vi "Publish (Raw Payload).vi"(4 "timeout (1000ms)":i32=1000, 5 "RETAIN":bool, 6 "QoS":T1, 7 "DUP (Re-delivery attempt)":bool, 8 "error in (no error)":errorcluster, 9 "Binary Payload":u8[](array[numeric]) format="%08b", 10 "Topic Name":string, 11 "Client in":refnum<class "Client.lvclass">) -> (0 "error out":errorcluster, 2 "Published":bool, 3 "Client out":refnum<class "Client.lvclass">)   [LabVIEW 2013, in "MQTT Client.lvlib" / "Client.lvclass"]
uses:
  Client.lvclass
  <vilib>/LabVIEW Open Source Project/MQTT Control Packets/Control Packets/ControlPacket/QualityOfService -- enum.ctl
  <vilib>/LabVIEW Open Source Project/MQTT Control Packets/Control Packets/PUBLISH/PUBLISH.lvclass
  <vilib>/LabVIEW Open Source Project/MQTT Control Packets/Control Packets/ControlPacket/ControlPacket.lvclass
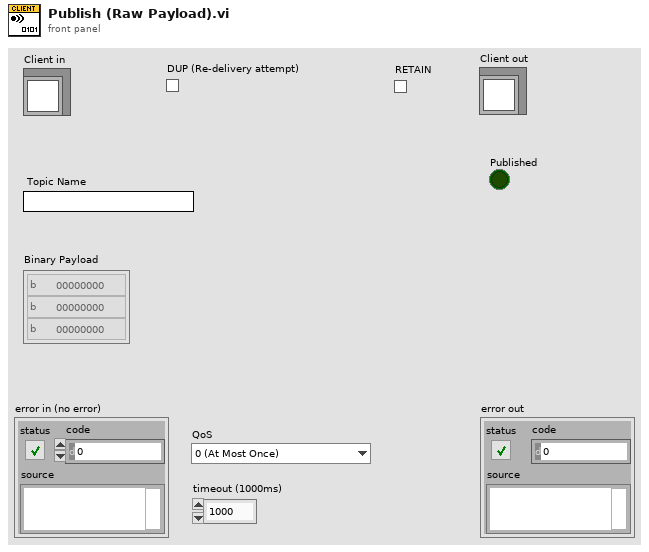
[diagram p1: front panel]
types:
  T1 = typedef "MQTT_Control_Packets.lvlib/ControlPacket.lvclass/QualityOfService -- enum.ctl" = enum16{"0 (At Most Once)", "1 (At Least Once)", "2 (Exactly Once)"}
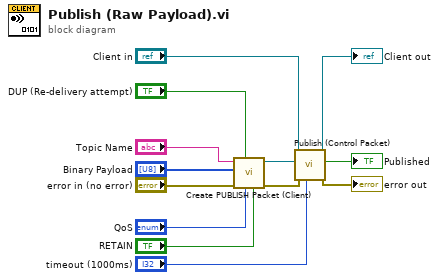
[diagram p0: block diagram]
diagram:
  n1 = call <vilib>:"Create PUBLISH Packet (Client).vi"("RETAIN"="RETAIN", "QoS"="QoS", "DUP (Re-delivery attempt)"="DUP (Re-delivery attempt)", "error in (no error)"="error in (no error)", "Payload"="Binary Payload", "Topic Name"="Topic Name") -> ("error out"=w3:errorcluster, "PUBLISH"=w4:refnum<class "PUBLISH.lvclass">)  [unwired: 2 in, 2 out]
  n2 = call "Publish (Control Packet).vi"("timeout (1000ms)"="timeout (1000ms)", "error in (no error)"=w3, "PUBLISH"=w4, "Client in"="Client in") -> ("error out"=→"error out":errorcluster, "Published"=→"Published":bool, "Client out"=→"Client out":refnum<class "Client.lvclass">)  [unwired: 5 in]
